vi "Convex Hull Test.vi"() -> ()   [LabVIEW 2018]
uses:
  Shared/Graham Scan/Graham Scan Point.ctl
  3d2dd41f-ec83-465a-86cd-b73e5684b592.vi
  665af295-381f-45f0-97ed-36c5abda909f.vi
  3d2dd41f-ec83-465a-86cd-b73e5684b592.vi/68ce29a8-b79f-41c8-8e39-aceefce0c8e0.vi
  665af295-381f-45f0-97ed-36c5abda909f.vi/9553dac6-d3a5-4753-b014-e5e4650516a4.vi
panel:
  out "Array":cluster{"X":dbl, "Y":dbl}[](array[cluster])
  out "Interior":cluster{"X":i32, "Y":i32}[](graph)
  out "Hull":cluster{"X":i32, "Y":i32}[](graph)
  out "Sorted":cluster{"X":i32, "Y":i32}[](graph)
  out "Scattered":cluster{"X":i32, "Y":i32}[](graph)
  in  "Number of Points":i32=100
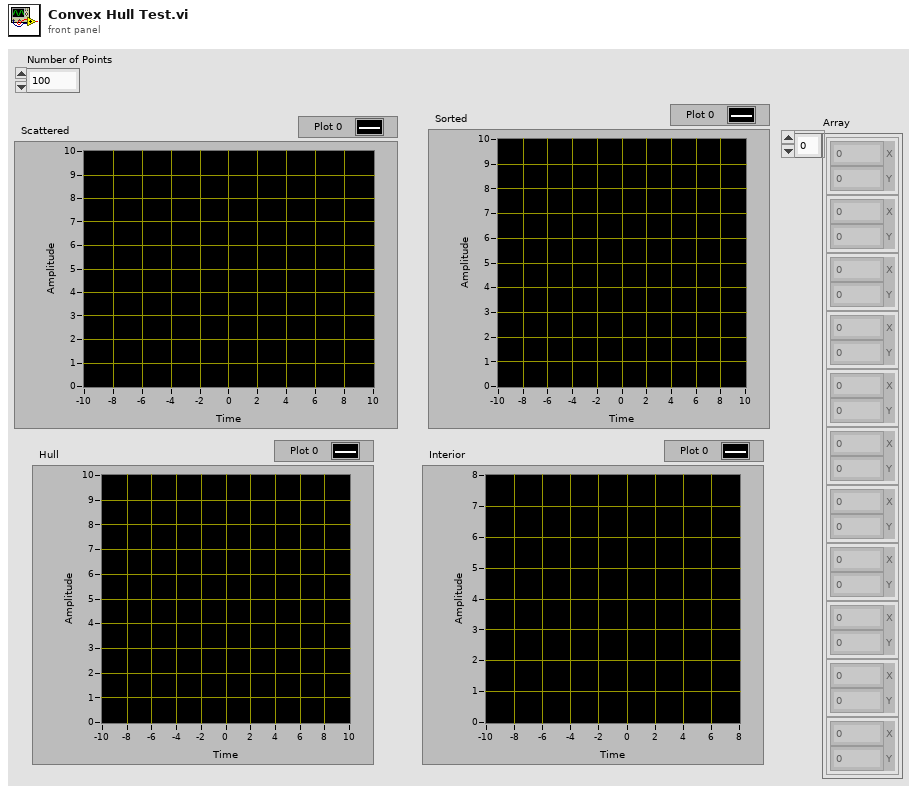
[diagram p1: front panel]
types:
  T1 = typedef "Graham Scan Point.ctl" = cluster{"X":i32, "Y":i32}
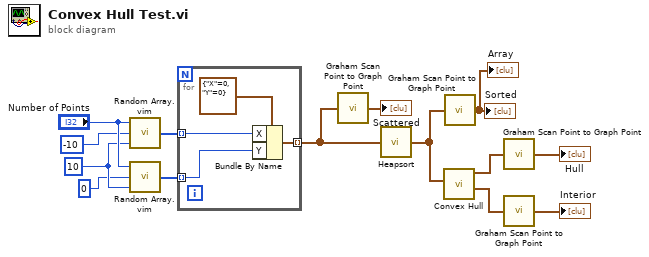
[diagram p0: block diagram]
diagram:
  w12 = 10
  n1 = call "Random Array.vim"("Max. (1, inc.)"=w12, "Min. (0, inc.)"=-10, "Number of Elements (100)"="Number of Points") -> ("Random Array"=w11:i32[])
  n2 = call "Random Array.vim"("Max. (1, inc.)"=w12, "Min. (0, inc.)"=0, "Number of Elements (100)"="Number of Points") -> ("Random Array"=w10:i32[])
  n3 = for {
    tunnel: w11 -> [w17] mode=indexing
    tunnel: w10 -> [w16] mode=indexing
    tunnel: [w15] -> w8 mode=indexing
    n4 = Bundle By Name(cluster=T1 {"X"=0, "Y"=0} ("Point"), "X"=w17, "Y"=w16) -> (w15:T1)
  }
  n5 = call "Graham Scan Point to Graph Point.vi"("Array"=w8) -> ("Array Out"=→"Scattered":cluster{"X":i32, "Y":i32}[])
  n6 = call "Heapsort.vi"("Array"=w8) -> ("Sorted Array"=w3:T1[])
  n7 = call "Convex Hull.vi"("Sorted Array"=w3) -> ("Interior Points"=w1:T1[], "Convex Hull"=w2:T1[])  [unwired: 5 in]
  n8 = call "Graham Scan Point to Graph Point.vi"("Array"=w3) -> ("Array Out"=→"Sorted" →"Array":cluster{"X":i32, "Y":i32}[])
  n9 = call "Graham Scan Point to Graph Point.vi"("Array"=w2) -> ("Array Out"=→"Hull":cluster{"X":i32, "Y":i32}[])
  n10 = call "Graham Scan Point to Graph Point.vi"("Array"=w1) -> ("Array Out"=→"Interior":cluster{"X":i32, "Y":i32}[])
